vi "test_VI Set-Get Protocol UDP.vi"(8 "error in (no error)":errorcluster, 11 "TestCase in":refnum<class "Instrument Addon Scripting API Custom Device Unit Tests.lvclass">) -> (0 "error out":errorcluster, 3 "TestCase out":refnum<class "Instrument Addon Scripting API Custom Device Unit Tests.lvclass">)   [LabVIEW 2018, in "Instrument Addon Scripting API Custom Device Unit Tests.lvclass"]
uses:
  Instrument Addon Scripting API Custom Device Unit Tests.lvclass
  Addon/Support Libraries/Protocols.lvlibp/UDP/UDP.lvclass
  C:/Users/nitest/Git/NI VS Instrument Addon Fork/Source/Addon/Support Libraries/Protocols.lvlibp/Protocol Parent/Protocol Parent.lvclass
  NationalInstruments.VeriStand.SystemDefinitionAPI
  Addon/Support Libraries/Protocols.lvlibp/UDP/Data Access/Write Local IP Address.vi
  Addon/Support Libraries/Protocols.lvlibp/UDP/Data Access/Write Local Port.vi
  Addon/Support Libraries/Protocols.lvlibp/UDP/Data Access/Write Target IP Address.vi
  Addon/Support Libraries/Protocols.lvlibp/UDP/Data Access/Write Target Port.vi
  Instrument Addon Scripting API Test Assets/Instrument Addon Scripting API Test Assets.lvclass
  <vilib>/addons/_JKI Toolkits/VI Tester/TestCase.llb/TestCase.lvclass
  APIs/Scripting API/Instrument Addon Scripting API.lvlib
  C:/Program Files (x86)/National Instruments/LabVIEW 2018/vi.lib/addons/_JKI Toolkits/VI Tester/TestCase.llb/TestCase.lvclass
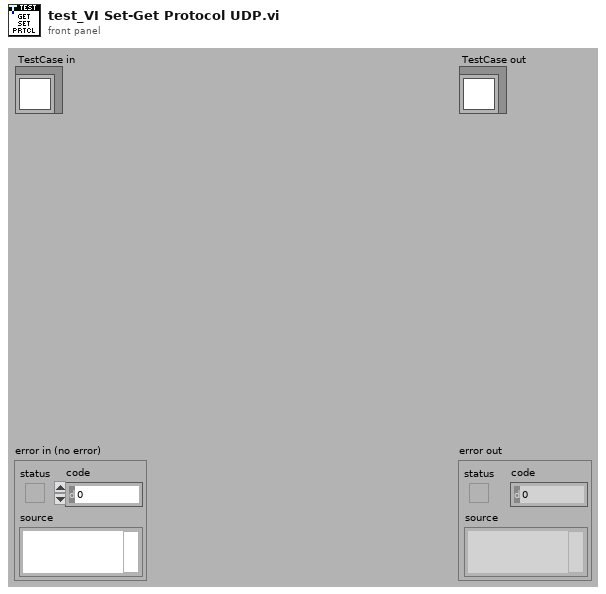
[diagram p1: front panel]
types:
  T1 = typedef "Custom Device API.lvlib/Custom Device Item Ref.ctl" = u64
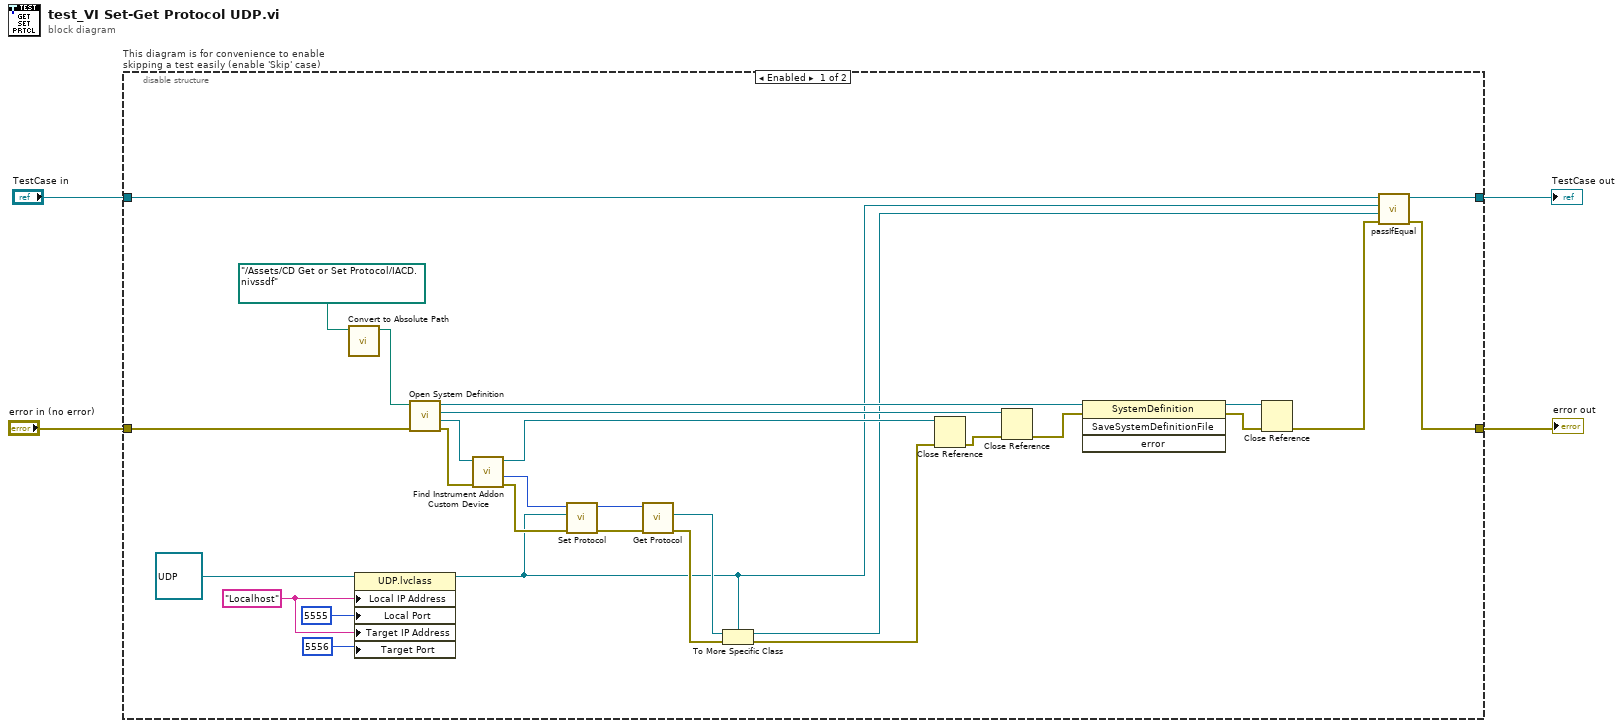
[diagram p0: block diagram]
diagram:
  n1 = disable-structure "This diagram is for convenience to enable skipping a test easily (enable 'Skip' case)" shown="Enabled" {
    disable-tunnel: "TestCase in" -> [w14 w37]
    disable-tunnel: [w13 w35] -> w1
    disable-tunnel: [w9 w36] -> w3
    disable-tunnel: "error in (no error)" -> [w33 w34]
    frame Enabled {
      w5 = "Localhost" ("VISA Resource")
      n2 = call "Convert to Absolute Path.vi"("System Definition File"=path "../Assets/CD Get or Set Protocol/IACD.nivssdf" ("SDF file")) -> ("Absolute Path"=w31:path)  [unwired: 10 in]
      n3 = property class="UDP.lvclass"(reference=refnum<class "UDP.lvclass"> refnum ("Protocols.lvlibp:UDP.lvclass"), "Local IP Address"=w5, "Local Port"=u16 5555, "Target IP Address"=w5, "Target Port"=u16 5556 ("Local Port")) -> (reference out=w11:refnum<class "UDP.lvclass">)  [unwired: 1 in, 1 out]
      n4 = call "Open System Definition.vi"("error in (no error)"=w33, "System Definition File"=w31) -> ("error out"=w28:errorcluster, "Target Refnum"=w27:refnum<k24>, "Root Refnum"=w30:refnum<k24>, "System Definition Refnum"=w21:refnum<k24>)  [unwired: 6 in]
      n5 = call "Find Instrument Addon Custom Device.vi"("error in"=w28, "target in"=w27) -> ("error out"=w26:errorcluster, "NodeID"=w25:u64, "target out"=w24:refnum<k24>)  [unwired: 7 in]
      n6 = call "Set Protocol.vi"("Error In"=w26, "Protocol in"=w11, "Instrument Addon Refnum In"=w25) -> ("Error Out"=w22:errorcluster, "Instrument Addon Refnum Out"=w23:T1)  [unwired: 7 in]
      n7 = call "Get Protocol.vi"("Error In"=w22, "Instrument Addon Refnum In"=w23) -> ("Error Out"=w16:errorcluster, "Protocol"=w17:refnum<class "Protocol Parent.lvclass">)  [unwired: 7 in, 1 out]
      n8 = To More Specific Class(target class=w11, reference=w17, error in=w16) -> (specific class reference=w12:refnum<class "UDP.lvclass">, error out=w15:errorcluster)
      n9 = Close Reference(reference=w24, error in (no error)=w15) -> (error out=w29:errorcluster)
      n10 = Close Reference(reference=w30, error in (no error)=w29) -> (error out=w20:errorcluster)
      n11 = invoke class="SystemDefinition" method="SaveSystemDefinitionFile"(reference=w21, error in=w20) -> (reference out=w19:refnum<k24>, error out=w18:errorcluster)  [unwired: 2 in, 2 out]
      n12 = Close Reference(reference=w19, error in (no error)=w18) -> (error out=w10:errorcluster)
      n13 = call-dynamic "passIfEqual.vi"("error in (no error)"=w10, "y"=w12, "x"=w11, "TestCase in"=w14) -> ("error out"=w9:errorcluster, "TestCase out"=w13:refnum<class "Instrument Addon Scripting API Custom Device Unit Tests.lvclass">)  [unwired: 6 in]
    }
    frame Disabled {
      # "skip test result while test is under development"
      n14 = call <vilib>:"skip.vi"("error in (no error)"=w34, "TestCase in"=w37) -> ("error out"=w36:errorcluster, "TestCase out"=w35:refnum<class "Instrument Addon Scripting API Custom Device Unit Tests.lvclass">)  [unwired: 8 in]
    }
  }
  "error out" <- w3
  "TestCase out" <- w1
